vi "Begin.vi"(8 "error in":errorcluster) -> (0 "error out":errorcluster, 2 "Outputs":T1={"West Coast Drive Dev-ref"={"DevStatus"={"status"=FALSE, "code"=0, "source"=""}, "Motors[]"=[], "Square Inputs"=FALSE, "Max Output"=1.0}, "Driver Gamepad"={"Device"=enum."USB 0"}, "Operator Gamepad"={"Device"=enum."USB 0"}, "Shifting Solenoid 1"={"DevStatus"={"status"=FALSE, "code"=0, "source"=""}, "Pneumatics Control Module"=0, "Forward Solenoid Channel"=enum."Invalid", "Reverse Solenoid Channel"=enum."Invalid"}, "Motors"={"Lift Motor 1"={"DeviceStatus"={"status"=FALSE, "code"=0, "source"=""}, "Type"=enum."PWM", "PWM"={"Controller"=enum."Controller 1", "PWM Channel"=enum."PWM 0", "DeadBand"={"Name"="", "maxPositivePwm"=0, "minPositivePwm"=0, "centerPwm"=0, "maxNegativePwm"=0, "minNegativePwm"=0, "angularRange"=0}}, "CAN"={"Device Number"=0, "Control Mode"=enum."Percent VBus", "Semaphore"=refnum, "Max Vout"=0.0, "TalonSRX Control Mode"=enum."Percent VBus"}, "Invert"=FALSE, "TransformRef"=refnum, "InvTransformRef"=refnum}, "Gripper Motor"={"DeviceStatus"={"status"=FALSE, "code"=0, "source"=""}, "Type"=enum."PWM", "PWM"={"Controller"=enum."Controller 1", "PWM Channel"=enum."PWM 0", "DeadBand"={"Name"="", "maxPositivePwm"=0, "minPositivePwm"=0, "centerPwm"=0, "maxNegativePwm"=0, "minNegativePwm"=0, "angularRange"=0}}, "CAN"={"Device Number"=0, "Control Mode"=enum."Percent VBus", "Semaphore"=refnum, "Max Vout"=0.0, "TalonSRX Control Mode"=enum."Percent VBus"}, "Invert"=FALSE, "TransformRef"=refnum, "InvTransformRef"=refnum}, "Lift Motor 2"={"DeviceStatus"={"status"=FALSE, "code"=0, "source"=""}, "Type"=enum."PWM", "PWM"={"Controller"=enum."Controller 1", "PWM Channel"=enum."PWM 0", "DeadBand"={"Name"="", "maxPositivePwm"=0, "minPositivePwm"=0, "centerPwm"=0, "maxNegativePwm"=0, "minNegativePwm"=0, "angularRange"=0}}, "CAN"={"Device Number"=0, "Control Mode"=enum."Percent VBus", "Semaphore"=refnum, "Max Vout"=0.0, "TalonSRX Control Mode"=enum."Percent VBus"}, "Invert"=FALSE, "TransformRef"=refnum, "InvTransformRef"=refnum}}, "Limit Switches"={"SwitchDevRef"={"DevStatus"={"status"=FALSE, "code"=0, "source"=""}, "DIO Channel"=enum."DIO 0", "Controller"=enum."Controller 1", "CntIndex"=enum."Ctr 0", "Normally Closed"=FALSE}, "SwitchDevRef 2"={"DevStatus"={"status"=FALSE, "code"=0, "source"=""}, "DIO Channel"=enum."DIO 0", "Controller"=enum."Controller 1", "CntIndex"=enum."Ctr 0", "Normally Closed"=FALSE}, "SwitchDevRef 3"={"DevStatus"={"status"=FALSE, "code"=0, "source"=""}, "DIO Channel"=enum."DIO 0", "Controller"=enum."Controller 1", "CntIndex"=enum."Ctr 0", "Normally Closed"=FALSE}, "SwitchDevRef 4"={"DevStatus"={"status"=FALSE, "code"=0, "source"=""}, "DIO Channel"=enum."DIO 0", "Controller"=enum."Controller 1", "CntIndex"=enum."Ctr 0", "Normally Closed"=FALSE}}, "Drive Encoders"={"EncoderDevRef"={"DevStatus"={"status"=FALSE, "code"=0, "source"=""}, "EncoderIndex"=enum."Enc 0", "CounterIndex"=enum."Ctr 0", "DistancePerCount"=0.0, "Decoding Type"=enum."1x"}, "EncoderDevRef"={"DevStatus"={"status"=FALSE, "code"=0, "source"=""}, "EncoderIndex"=enum."Enc 0", "CounterIndex"=enum."Ctr 0", "DistancePerCount"=0.0, "Decoding Type"=enum."1x"}}, "Gripper Encoder"={"DevStatus"={"status"=FALSE, "code"=0, "source"=""}, "EncoderIndex"=enum."Invalid", "CounterIndex"=enum."Invalid", "DistancePerCount"=1.0, "Decoding Type"=enum."4x"}, "Lift Potentiometer"={"DevStatus"={"status"=FALSE, "code"=0, "source"=""}, "Controller"=enum."Controller 1", "Analog Channel"=enum."Invalid", "Invert Output"=FALSE}, "Shifting Solenoid 2"={"DevStatus"={"status"=FALSE, "code"=0, "source"=""}, "Pneumatics Control Module"=0, "Forward Solenoid Channel"=enum."Invalid", "Reverse Solenoid Channel"=enum."Invalid"}, "Gyro"={"DevStatus"={"status"=FALSE, "code"=0, "source"=""}, "Analog Module"=enum."Controller 1", "Analog Channel"=enum."AI 1", "Offset"=0.0, "Gain (VoltsPerDegree/Second)"=0.0}, "Buttons"={"Device"=enum."USB 0"}})   [LabVIEW 2014]
doc: "Called before other user functions, this VI is expected to open initial I/O refnums, load in file data, and do all program initialization. Notice that the <B>error out</B> terminal is simply used for data flow. Wiring it to other structures or subVIs ensures that this VI runs first."
uses:
  SubVI/cluster data.ctl
  <vilib>/Rock Robotics/WPI/RobotDrive/WPI_RobotDriveDevRef.ctl
  <vilib>/Rock Robotics/WPI/MotorControl/WPI_MotorControlDeviceRef.ctl
  <vilib>/Rock Robotics/WPI/MotorControl/WPI_MotorControlType.ctl
  <vilib>/Rock Robotics/SystemInterfaces/Typedef/FPGA_TypedefDigitalModule.ctl
  <vilib>/Rock Robotics/SystemInterfaces/DIO/FPGA_DIOPWMChannel.ctl
  <vilib>/Rock Robotics/WPI/PWM/WPI_PWMDeadband.ctl
  <vilib>/Rock Robotics/WPI/CAN/Jaguar/SubVIs/WPI_CANJaguar_ControlMode.ctl
  <vilib>/Rock Robotics/WPI/CAN/TalonSRX/WPI_CANTalonSRX_APIControlMode.ctl
  <vilib>/Rock Robotics/WPI/PWM/WPI_PWMTransform_ConPane.ctl
  <vilib>/Rock Robotics/WPI/Joystick/WPI_JoystickDevRef.ctl
  <vilib>/Rock Robotics/WPI/Joystick/WPI_JoystickDeviceEnum.ctl
  <vilib>/Rock Robotics/WPI/Solenoid/WPI_SolenoidDevRef.ctl
  <vilib>/Rock Robotics/WPI/Solenoid/WPI_SolenoidChannel.ctl
  <vilib>/Rock Robotics/WPI/Switch/WPI_SwitchDevRef.ctl
  <vilib>/Rock Robotics/SystemInterfaces/DIO/FPGA_DIOChannel.ctl
  <vilib>/Rock Robotics/SystemInterfaces/Counter/FPGA_CounterCtrSystemIndex.ctl
  <vilib>/Rock Robotics/WPI/Encoder/WPI_EncoderDevRef.ctl
  <vilib>/Rock Robotics/SystemInterfaces/Encoder/FPGA_EncoderIdx.ctl
  <vilib>/Rock Robotics/WPI/Encoder/WPI_EncoderType.ctl
  <vilib>/Rock Robotics/WPI/Potentiometer/WPI_PotentiometerDevRef.ctl
  <vilib>/Rock Robotics/SystemInterfaces/Typedef/FPGA_TypedefAnalogModule.ctl
  <vilib>/Rock Robotics/SystemInterfaces/AI/FPGA_AIChannel.ctl
  <vilib>/Rock Robotics/WPI/Gyro/WPI_GyroDevRef.ctl
  <vilib>/Rock Robotics/WPI/DriverStation/WPI_DriverStationRobotMode2.ctl
  <vilib>/Rock Robotics/SystemInterfaces/AI/FPGA_AIGyroChannel.ctl
  Robot Global Data.vi
  <vilib>/Rock Robotics/WPI/RobotDrive/WPI_RobotDriveOpen4MotorWithTalon.vi
  <vilib>/Rock Robotics/WPI/Solenoid/WPI_SolenoidOpenSingle.vi
  <vilib>/Rock Robotics/WPI/Counter/WPI_CounterDigitalInputToDigitalSource.vi
  <vilib>/Rock Robotics/WPI/Switch/WPI_SwitchOpenLimit.vi
  <vilib>/Rock Robotics/WPI/MotorControl/WPI_MotorControlOpen Talon.vi
  <vilib>/Rock Robotics/WPI/MotorControl/WPI_MotorControlOpenCANTalonSRX.vi
panel:
  in  "Begin outputs":T1={"West Coast Drive Dev-ref"={"DevStatus"={"status"=FALSE, "code"=0, "source"=""}, "Motors[]"=[], "Square Inputs"=FALSE, "Max Output"=1.0}, "Driver Gamepad"={"Device"=enum."USB 0"}, "Operator Gamepad"={"Device"=enum."USB 0"}, "Shifting Solenoid 1"={"DevStatus"={"status"=FALSE, "code"=0, "source"=""}, "Pneumatics Control Module"=0, "Forward Solenoid Channel"=enum."Invalid", "Reverse Solenoid Channel"=enum."Invalid"}, "Motors"={"Lift Motor 1"={"DeviceStatus"={"status"=FALSE, "code"=0, "source"=""}, "Type"=enum."PWM", "PWM"={"Controller"=enum."Controller 1", "PWM Channel"=enum."Invalid", "DeadBand"={"Name"="", "maxPositivePwm"=0, "minPositivePwm"=0, "centerPwm"=0, "maxNegativePwm"=0, "minNegativePwm"=0, "angularRange"=0}}, "CAN"={"Device Number"=0, "Control Mode"=enum."Percent VBus", "Semaphore"=refnum, "Max Vout"=12.0, "TalonSRX Control Mode"=enum."Percent VBus"}, "Invert"=FALSE, "TransformRef"=refnum, "InvTransformRef"=refnum}, "Gripper Motor"={"DeviceStatus"={"status"=FALSE, "code"=0, "source"=""}, "Type"=enum."PWM", "PWM"={"Controller"=enum."Controller 1", "PWM Channel"=enum."PWM 0", "DeadBand"={"Name"="", "maxPositivePwm"=0, "minPositivePwm"=0, "centerPwm"=0, "maxNegativePwm"=0, "minNegativePwm"=0, "angularRange"=0}}, "CAN"={"Device Number"=0, "Control Mode"=enum."Percent VBus", "Semaphore"=refnum, "Max Vout"=0.0, "TalonSRX Control Mode"=enum."Percent VBus"}, "Invert"=FALSE, "TransformRef"=refnum, "InvTransformRef"=refnum}, "Lift Motor 2"={"DeviceStatus"={"status"=FALSE, "code"=0, "source"=""}, "Type"=enum."PWM", "PWM"={"Controller"=enum."Controller 1", "PWM Channel"=enum."PWM 0", "DeadBand"={"Name"="", "maxPositivePwm"=0, "minPositivePwm"=0, "centerPwm"=0, "maxNegativePwm"=0, "minNegativePwm"=0, "angularRange"=0}}, "CAN"={"Device Number"=0, "Control Mode"=enum."Percent VBus", "Semaphore"=refnum, "Max Vout"=0.0, "TalonSRX Control Mode"=enum."Percent VBus"}, "Invert"=FALSE, "TransformRef"=refnum, "InvTransformRef"=refnum}}, "Limit Switches"={"SwitchDevRef"={"DevStatus"={"status"=FALSE, "code"=0, "source"=""}, "DIO Channel"=enum."DIO 0", "Controller"=enum."Controller 1", "CntIndex"=enum."Ctr 0", "Normally Closed"=FALSE}, "SwitchDevRef 2"={"DevStatus"={"status"=FALSE, "code"=0, "source"=""}, "DIO Channel"=enum."DIO 0", "Controller"=enum."Controller 1", "CntIndex"=enum."Ctr 0", "Normally Closed"=FALSE}, "SwitchDevRef 3"={"DevStatus"={"status"=FALSE, "code"=0, "source"=""}, "DIO Channel"=enum."DIO 0", "Controller"=enum."Controller 1", "CntIndex"=enum."Ctr 0", "Normally Closed"=FALSE}, "SwitchDevRef 4"={"DevStatus"={"status"=FALSE, "code"=0, "source"=""}, "DIO Channel"=enum."DIO 0", "Controller"=enum."Controller 1", "CntIndex"=enum."Ctr 0", "Normally Closed"=FALSE}}, "Drive Encoders"={"EncoderDevRef"={"DevStatus"={"status"=FALSE, "code"=0, "source"=""}, "EncoderIndex"=enum."Enc 0", "CounterIndex"=enum."Ctr 0", "DistancePerCount"=0.0, "Decoding Type"=enum."1x"}, "EncoderDevRef"={"DevStatus"={"status"=FALSE, "code"=0, "source"=""}, "EncoderIndex"=enum."Enc 0", "CounterIndex"=enum."Ctr 0", "DistancePerCount"=0.0, "Decoding Type"=enum."1x"}}, "Gripper Encoder"={"DevStatus"={"status"=FALSE, "code"=0, "source"=""}, "EncoderIndex"=enum."Invalid", "CounterIndex"=enum."Invalid", "DistancePerCount"=1.0, "Decoding Type"=enum."4x"}, "Lift Potentiometer"={"DevStatus"={"status"=FALSE, "code"=0, "source"=""}, "Controller"=enum."Controller 1", "Analog Channel"=enum."Invalid", "Invert Output"=FALSE}, "Shifting Solenoid 2"={"DevStatus"={"status"=FALSE, "code"=0, "source"=""}, "Pneumatics Control Module"=0, "Forward Solenoid Channel"=enum."Invalid", "Reverse Solenoid Channel"=enum."Invalid"}, "Gyro"={"DevStatus"={"status"=FALSE, "code"=0, "source"=""}, "Analog Module"=enum."Controller 1", "Analog Channel"=enum."AI 1", "Offset"=0.0, "Gain (VoltsPerDegree/Second)"=0.0}, "Buttons"={"Device"=enum."USB 0"}}
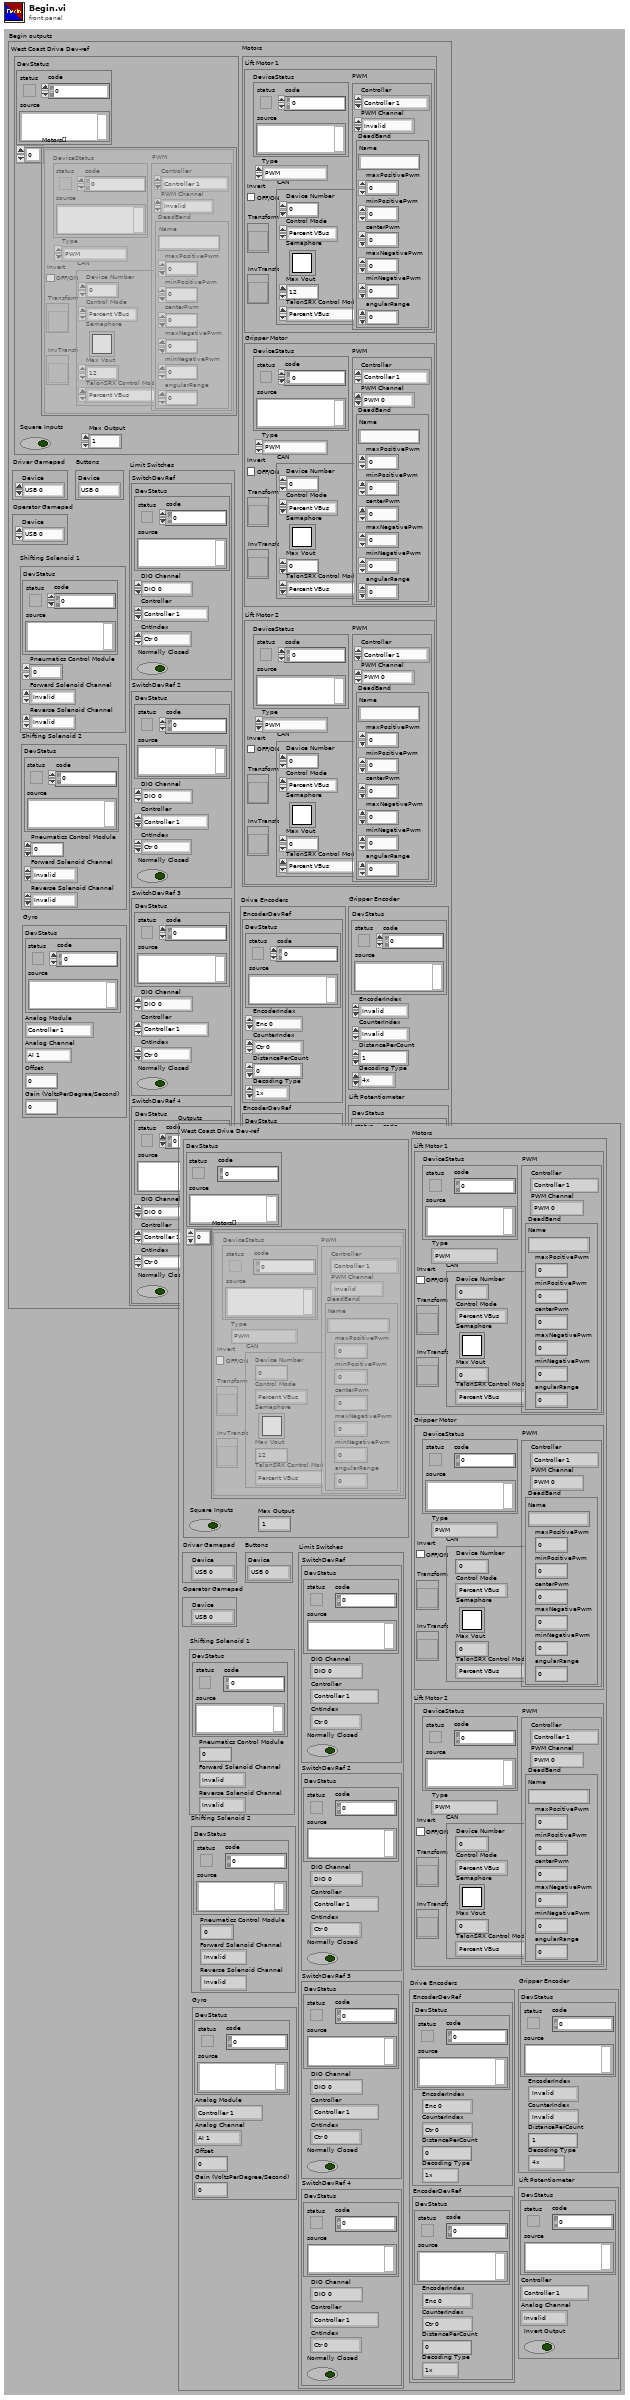
[diagram p1: front panel]
types:
  T1 = typedef "cluster data.ctl" = cluster{"West Coast Drive Dev-ref":T2, "Driver Gamepad":T12, "Operator Gamepad":T12, "Shifting Solenoid 1":T14, "Motors":cluster{"Lift Motor 1":T3, "Gripper Motor":T3, "Lift Motor 2":T3}, "Limit Switches":cluster{"SwitchDevRef":T16, "SwitchDevRef 2":T16, "SwitchDevRef 3":T16, "SwitchDevRef 4":T16}, "Drive Encoders":cluster{"EncoderDevRef":T19, "EncoderDevRef":T19}, "Gripper Encoder":T19, "Lift Potentiometer":T22, "Shifting Solenoid 2":T14, "Gyro":T25, "Buttons":T12}
  T2 = typedef "WPI_RobotDriveDevRef.ctl" = cluster{"DevStatus":errorcluster, "Motors[]":T3[], "Square Inputs":bool, "Max Output":dbl}
  T3 = typedef "WPI_MotorControlDeviceRef.ctl" = cluster{"DeviceStatus":errorcluster, "Type":T4, "PWM":cluster{"Controller":T5, "PWM Channel":T6, "DeadBand":T7}, "CAN":cluster{"Device Number":u8, "Control Mode":T8, "Semaphore":T9, "Max Vout":dbl, "TalonSRX Control Mode":T10}, "Invert":bool, "TransformRef":T11, "InvTransformRef":T11}
  T4 = typedef "WPI_MotorControlType.ctl" = enum16{"PWM", "CAN", "CANTalonSRX"}
  T5 = typedef "FPGA_TypedefDigitalModule.ctl" = enum16{"Controller 1"}
  T6 = typedef "FPGA_DIOPWMChannel.ctl" = enum8{"PWM 0", "PWM 1", "PWM 2", "PWM 3", "PWM 4", "PWM 5", "PWM 6", "PWM 7", "PWM 8", "PWM 9", "PWM MXP 0", "PWM MXP 1", "PWM MXP 2", "PWM MXP 3", "PWM MXP 4", "PWM MXP 5", "PWM MXP 6", "PWM MXP 7", "PWM MXP 8", "PWM MXP 9", "Invalid"}
  T7 = typedef "WPI_PWMDeadband.ctl" = cluster{"Name":string, "maxPositivePwm":i32, "minPositivePwm":i32, "centerPwm":i32, "maxNegativePwm":i32, "minNegativePwm":i32, "angularRange":u16}
  T8 = typedef "WPI_CANJaguar_ControlMode.ctl" = enum8{"Percent VBus", "Current", "Speed", "Position", "Voltage"}
  T9 = typedef "Semaphore RefNum" = refnum<k1>
  T10 = typedef "WPI_CANTalonSRX_APIControlMode.ctl" = enum8{"Percent VBus", "Speed", "Position", "Slave", "Unchanged / Invalid"}
  T11 = typedef "WPI_PWMTransform_ConPane.ctl" = refnum<vi>
  T12 = typedef "WPI_JoystickDevRef.ctl" = cluster{"Device":T13}
  T13 = typedef "WPI_JoystickDeviceEnum.ctl" = enum16{"USB 0", "USB 1", "USB 2", "USB 3", "USB 4", "USB 5"}
  T14 = typedef "WPI_SolenoidDevRef.ctl" = cluster{"DevStatus":errorcluster, "Pneumatics Control Module":u8, "Forward Solenoid Channel":T15, "Reverse Solenoid Channel":T15}
  T15 = typedef "WPI_SolenoidChannel.ctl" = enum8{"Solenoid 0", "Solenoid 1", "Solenoid 2", "Solenoid 3", "Solenoid 4", "Solenoid 5", "Solenoid 6", "Solenoid 7", "Invalid"}
  T16 = typedef "WPI_SwitchDevRef.ctl" = cluster{"DevStatus":errorcluster, "DIO Channel":T17, "Controller":T5, "CntIndex":T18, "Normally Closed":bool}
  T17 = typedef "FPGA_DIOChannel.ctl" = enum8{"DIO 0", "DIO 1", "DIO 2", "DIO 3", "DIO 4", "DIO 5", "DIO 6", "DIO 7", "DIO 8", "DIO 9", "DIO MXP 0", "DIO MXP 1", "DIO MXP 2", "DIO MXP 3", "DIO MXP 4", "DIO MXP 5", "DIO MXP 6", "DIO MXP 7", "DIO MXP 8", "DIO MXP 9", "DIO MXP 10", "DIO MXP 11", "DIO MXP 12", "DIO MXP 13", "DIO MXP 14", "DIO MXP 15", "Invalid"}
  T18 = typedef "FPGA_CounterCtrSystemIndex.ctl" = enum8{"Ctr 0", "Ctr 1", "Ctr 2", "Ctr 3", "Ctr 4", "Ctr 5", "Ctr 6", "Ctr 7", "Invalid"}
  T19 = typedef "WPI_EncoderDevRef.ctl" = cluster{"DevStatus":errorcluster, "EncoderIndex":T20, "CounterIndex":T18, "DistancePerCount":dbl, "Decoding Type":T21}
  T20 = typedef "FPGA_EncoderIdx.ctl" = enum8{"Enc 0", "Enc 1", "Enc 2", "Enc 3", "Enc 4", "Enc 5", "Enc 6", "Enc 7", "Invalid"}
  T21 = typedef "WPI_EncoderType.ctl" = enum16{"1x", "2x", "4x"}
  T22 = typedef "WPI_PotentiometerDevRef.ctl" = cluster{"DevStatus":errorcluster, "Controller":T23, "Analog Channel":T24, "Invert Output":bool}
  T23 = typedef "FPGA_TypedefAnalogModule.ctl" = enum16{"Controller 1"}
  T24 = typedef "FPGA_AIChannel.ctl" = enum8{"AI 0", "AI 1", "AI 2", "AI 3", "AI MXP 0", "AI MXP 1", "AI MXP 2", "AI MXP 3", "Invalid"}
  T25 = typedef "WPI_GyroDevRef.ctl" = cluster{"DevStatus":errorcluster, "Analog Module":T23, "Analog Channel":T24, "Offset":dbl, "Gain (VoltsPerDegree/Second)":dbl}
  T26 = cluster{"Lift Top":T16, "Lift Bottom":T16, "Gripper 1":T16, "Gripper 2":T16}
  T27 = typedef "FPGA_AIGyroChannel.ctl" = enum8{"AI 0", "AI 1", "Invalid"}
  T28 = typedef "WPI_DriverStationRobotMode2.ctl" = enum16{"Autonomous Disabled", "Autonomous Enabled", "Teleop Disabled", "Teleop Enabled", "Disconnected", "Finish", "Test Disabled", "Test Enabled", "Emergency Stopped"}
  T29 = typedef "WPI_DigitalInputDevRef.ctl" = cluster{"DevStatus":errorcluster, "DIO Channel":T17, "Controller":T5}
  T30 = typedef "FPGA_CounterEncoderSourceConvertionLVSourceType.ctl" = cluster{"DevStatus":errorcluster, "AnalogTriggerMode?":bool, "DigitalMode":cluster{"Controller":T5, "DIO Channel":T31}, "AnalogTriggerMode":cluster{"AnalogTriggerIndex":T32, "OutputType":T33}}
  T31 = typedef "FPGA_DIODigitalSourceChannel.ctl" = enum8{"DIO 0", "DIO 1", "DIO 2", "DIO 3", "DIO 4", "DIO 5", "DIO 6", "DIO 7", "DIO 8", "DIO 9", "DIO MXP 0", "DIO MXP 1", "DIO MXP 2", "DIO MXP 3", "DIO MXP 4", "DIO MXP 5", "DIO MXP 6", "DIO MXP 7", "DIO MXP 8", "DIO MXP 9", "DIO MXP 10", "DIO MXP 11", "DIO MXP 12", "DIO MXP 13", "DIO MXP 14", "DIO MXP 15", "Disabled"}
  T32 = typedef "FPGA_AnalogTriggerIndex.ctl" = enum8{"Trig 0", "Trig 1", "Trig 2", "Trig 3", "Trig 4", "Trig 5", "Trig 6", "Trig 7", "Invalid"}
  T33 = typedef "FPGA_AnalogTriggerOutType.ctl" = enum16{"InWindow", "TriggerState", "Rising", "Falling"}
  T34 = cluster{"EncoderDevRef":T19, "EncoderDevRef":T19}
  T35 = cluster{"MotorControlDeviceRef":T3, "MotorControlDeviceRef":T3, "MotorControlDeviceRef":T3}
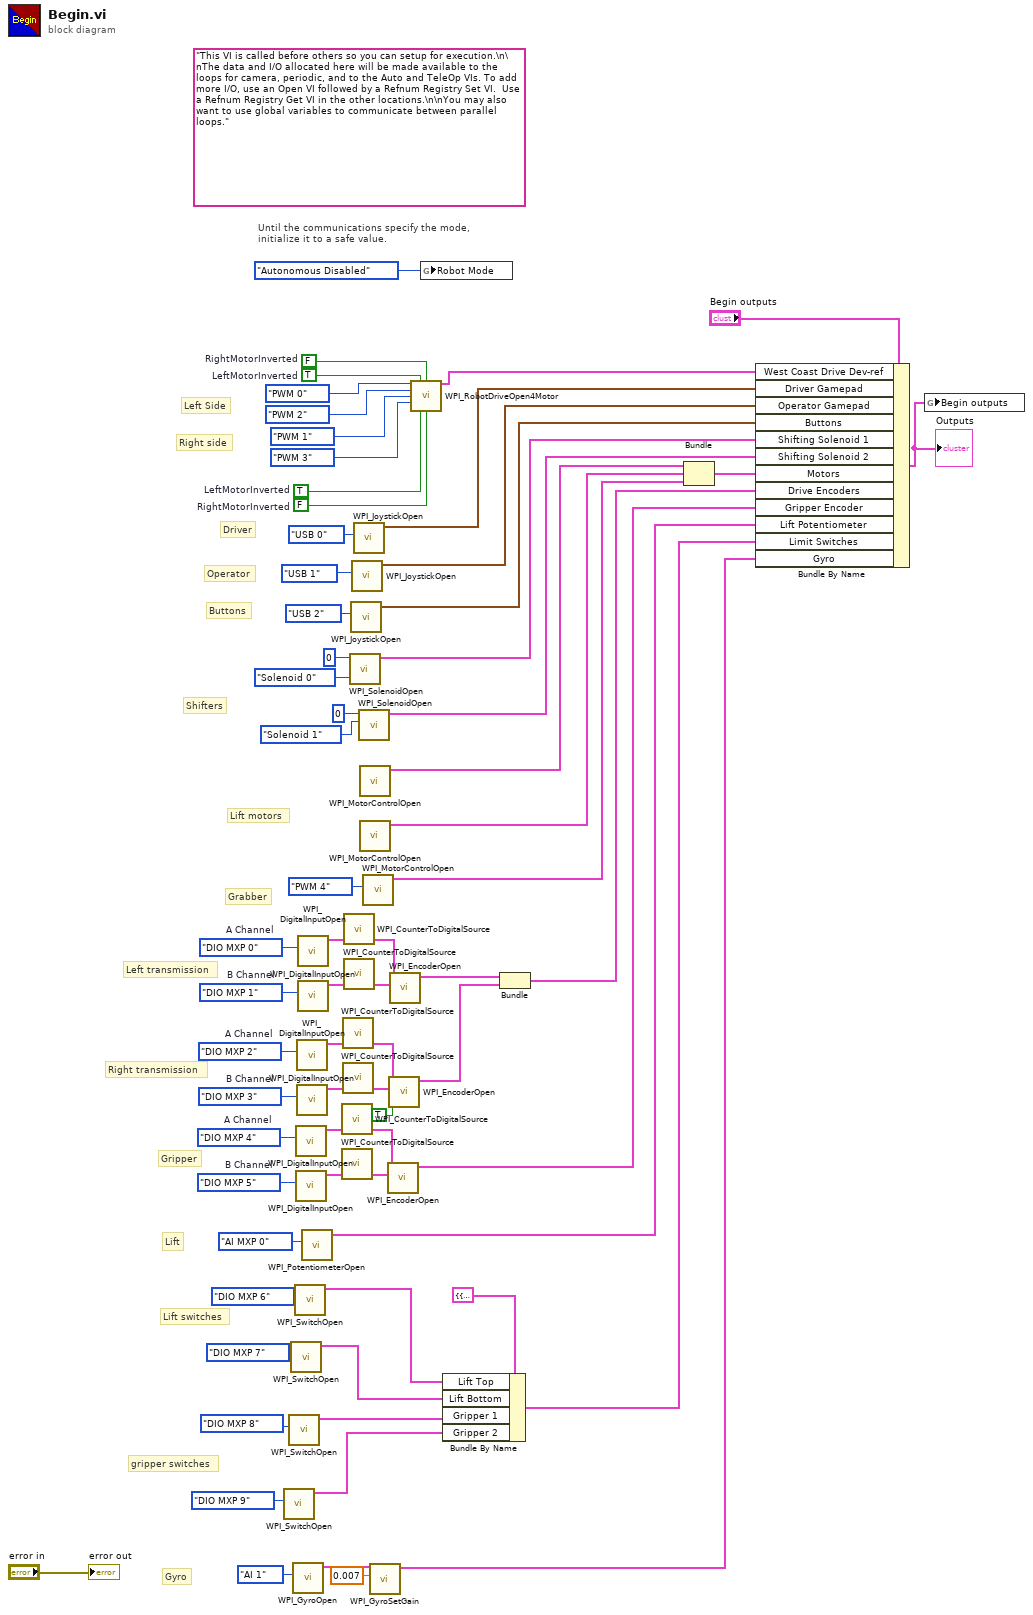
[diagram p0: block diagram]
diagram:
  w36 = FPGA_DIOChannel."DIO MXP 5"  # B Channel
  w35 = FPGA_DIOChannel."DIO MXP 4"  # A Channel
  w42 = FPGA_DIOChannel."DIO MXP 3"  # B Channel
  w41 = FPGA_DIOChannel."DIO MXP 2"  # A Channel
  w48 = FPGA_DIOChannel."DIO MXP 1"  # B Channel
  w47 = FPGA_DIOChannel."DIO MXP 0"  # A Channel
  w61 = FALSE  # RightMotorInverted
  w60 = TRUE  # LeftMotorInverted
  (unwired) "This VI is called before others so you can setup for execution.\n\nThe data and I/O allocated here will be made available to the loops for camera, periodic, and to the Auto and TeleOp VIs. To add more I/O, use an Open VI followed by a Refnum Registry Set VI.  Use a Refnum Registry Get VI in the other locations.\n\nYou may also want to use global variables to communicate between parallel loops."
  w67 = TRUE  # LeftMotorInverted
  w66 = FALSE  # RightMotorInverted
  # "Buttons"
  # "Gyro"
  # "gripper switches"
  # "Lift switches"
  # "Gripper"
  # "Lift"
  # "Right transmission"
  # "Left transmission"
  # "Grabber"
  # "Lift motors"
  # "Shifters"
  # "Operator"
  # "Driver"
  # "Right side"
  # "Left Side"
  # "Until the communications specify the mode,\ninitialize it to a safe value."
  n1 = call-poly <vilib>:"WPI_SwitchOpen.vi"("DIO Channel"=FPGA_DIOChannel."DIO MXP 9") -> ("SwitchDevRef"=w22:T16)  [unwired: 9 in, 1 out]
  n2 = call-poly <vilib>:"WPI_SwitchOpen.vi"("DIO Channel"=FPGA_DIOChannel."DIO MXP 8") -> ("SwitchDevRef"=w16:T16)  [unwired: 9 in, 1 out]
  n3 = call-poly <vilib>:"WPI_SwitchOpen.vi"("DIO Channel"=FPGA_DIOChannel."DIO MXP 7") -> ("SwitchDevRef"=w23:T16)  [unwired: 9 in, 1 out]
  n4 = call <vilib>:"WPI_GyroOpen.vi"("Analog Channel"=FPGA_AIGyroChannel."AI 1") -> ("GyroDevRef"=w5:T25)  [unwired: 8 in, 2 out]
  n5 = call-poly <vilib>:"WPI_SwitchOpen.vi"("DIO Channel"=FPGA_DIOChannel."DIO MXP 6") -> ("SwitchDevRef"=w24:T16)  [unwired: 9 in, 1 out]
  n6 = call <vilib>:"WPI_DigitalInputOpen.vi"("DIO Channel"=w35) -> ("DigitalInputDevRef"=w32:T29)  [unwired: 2 in, 8 out]
  n7 = call <vilib>:"WPI_DigitalInputOpen.vi"("DIO Channel"=w36) -> ("DigitalInputDevRef"=w33:T29)  [unwired: 2 in, 8 out]
  n8 = call <vilib>:"WPI_DigitalInputOpen.vi"("DIO Channel"=w41) -> ("DigitalInputDevRef"=w38:T29)  [unwired: 2 in, 8 out]
  n9 = call <vilib>:"WPI_DigitalInputOpen.vi"("DIO Channel"=w42) -> ("DigitalInputDevRef"=w39:T29)  [unwired: 2 in, 8 out]
  n10 = call <vilib>:"WPI_DigitalInputOpen.vi"("DIO Channel"=w47) -> ("DigitalInputDevRef"=w44:T29)  [unwired: 2 in, 8 out]
  n11 = call <vilib>:"WPI_DigitalInputOpen.vi"("DIO Channel"=w48) -> ("DigitalInputDevRef"=w45:T29)  [unwired: 2 in, 8 out]
  n12 = call <vilib>:"WPI_PotentiometerOpen.vi"("Analog Channel"=FPGA_AIChannel."AI MXP 0") -> ("PotDevRef"=w17:T22)  [unwired: 9 in, 1 out]
  n13 = call-poly <vilib>:"WPI_CounterToDigitalSource.vi"("DigitalInputDevRef"=w32) -> ("Digital Source"=w31:T30)  [unwired: 6 out]
  n14 = call-poly <vilib>:"WPI_CounterToDigitalSource.vi"("DigitalInputDevRef"=w33) -> ("Digital Source"=w34:T30)  [unwired: 6 out]
  n15 = call-poly <vilib>:"WPI_CounterToDigitalSource.vi"("DigitalInputDevRef"=w38) -> ("Digital Source"=w37:T30)  [unwired: 6 out]
  n16 = call-poly <vilib>:"WPI_CounterToDigitalSource.vi"("DigitalInputDevRef"=w39) -> ("Digital Source"=w40:T30)  [unwired: 6 out]
  n17 = call-poly <vilib>:"WPI_CounterToDigitalSource.vi"("DigitalInputDevRef"=w44) -> ("Digital Source"=w43:T30)  [unwired: 6 out]
  n18 = call-poly <vilib>:"WPI_CounterToDigitalSource.vi"("DigitalInputDevRef"=w45) -> ("Digital Source"=w46:T30)  [unwired: 6 out]
  n19 = call-poly <vilib>:"WPI_SolenoidOpen.vi"("Solenoid Channel"=WPI_SolenoidChannel."Solenoid 0" ("Forward Solenoid Channel"), "Pneumatics Control Module (0)"=u8 0) -> ("SolenoidDevRef"=w52:T14)  [unwired: 8 in, 1 out]
  n20 = call <vilib>:"WPI_JoystickOpen.vi"("JoystickDevice"=WPI_JoystickDeviceEnum."USB 2") -> ("JoystickDevRef"=w1:T12)  [unwired: 10 in]
  n21 = call <vilib>:"WPI_JoystickOpen.vi"("JoystickDevice"=WPI_JoystickDeviceEnum."USB 1") -> ("JoystickDevRef"=w58:T12)  [unwired: 10 in]
  n22 = call <vilib>:"WPI_JoystickOpen.vi"("JoystickDevice"=WPI_JoystickDeviceEnum."USB 0") -> ("JoystickDevRef"=w57:T12)  [unwired: 10 in]
  n23 = call-poly <vilib>:"WPI_SolenoidOpen.vi"("Solenoid Channel"=WPI_SolenoidChannel."Solenoid 1" ("Reverse Solenoid Channel"), "Pneumatics Control Module (0)"=u8 0) -> ("SolenoidDevRef"=w12:T14)  [unwired: 8 in, 1 out]
  n24 = call-poly <vilib>:"WPI_MotorControlOpen.vi"() -> ("MotorControlDeviceRef"=w50:T3)  [unwired: 10 in, 1 out]
  n25 = call-poly <vilib>:"WPI_MotorControlOpen.vi"() -> ("MotorControlDeviceRef"=w49:T3)  [unwired: 10 in, 1 out]
  n26 = call-poly <vilib>:"WPI_MotorControlOpen.vi"("PWM Channel"=FPGA_DIOPWMChannel."PWM 4") -> ("MotorControlDeviceRef"=w8:T3)  [unwired: 9 in, 1 out]
  n27 = call <vilib>:"WPI_GyroSetGain.vi"("Gain (VoltsPerDegree/Second)"=0.007, "GyroDevRef"=w5) -> ("GyroDevRef"=w4:T25)  [unwired: 8 in, 1 out]
  n28 = call <vilib>:"WPI_EncoderOpen.vi"("BSource"=w34, "ASource"=w31) -> ("EncoderDevRef"=w18:T19)  [unwired: 6 in, 3 out]
  n29 = call <vilib>:"WPI_EncoderOpen.vi"("Invert Direction (False)"=TRUE, "BSource"=w40, "ASource"=w37) -> ("EncoderDevRef"=w20:T19)  [unwired: 5 in, 3 out]
  n30 = call <vilib>:"WPI_EncoderOpen.vi"("BSource"=w46, "ASource"=w43) -> ("EncoderDevRef"=w21:T19)  [unwired: 6 in, 3 out]
  n31 = call-poly <vilib>:"WPI_RobotDriveOpen4Motor.vi"("Rear Left Motor"=FPGA_DIOPWMChannel."PWM 0", "Rear Left Motor Inverted"=w67, "Rear Right Motor Inverted"=w66, "Rear Right Motor"=FPGA_DIOPWMChannel."PWM 2", "Front Left Motor"=FPGA_DIOPWMChannel."PWM 1", "Front Right Motor"=FPGA_DIOPWMChannel."PWM 3", "Front Left Motor Inverted"=w60, "Front Right Motor Inverted"=w61) -> ("RobotDriveDevRef"=w59:T2)  [unwired: 6 in, 1 out]
  n32 = global write "Robot Global Data.vi" "Robot Mode"(WPI_DriverStationRobotMode2."Autonomous Disabled" ("Robot Mode")) -> ()
  n33 = Bundle By Name(cluster=T26 {"Lift Top"={"DevStatus"={"status"=FALSE, "code"=0, "source"=""}, "DIO Channel"=enum."Invalid", "Controller"=enum."Controller 1", "CntIndex"=enum."Invalid", "Normally Closed"=FALSE}, "Lift Bottom"={"DevStatus"={"status"=FALSE, "code"=0, "source"=""}, "DIO Channel"=enum."Invalid", "Controller"=enum."Controller 1", "CntIndex"=enum."Invalid", "Normally Closed"=FALSE}, "Gripper 1"={"DevStatus"={"status"=FALSE, "code"=0, "source"=""}, "DIO Channel"=enum."Invalid", "Controller"=enum."Controller 1", "CntIndex"=enum."Invalid", "Normally Closed"=FALSE}, "Gripper 2"={"DevStatus"={"status"=FALSE, "code"=0, "source"=""}, "DIO Channel"=enum."Invalid", "Controller"=enum."Controller 1", "CntIndex"=enum."Invalid", "Normally Closed"=FALSE}} ("Limit Switches"), "Lift Top"=w24, "Lift Bottom"=w23, "Gripper 1"=w16, "Gripper 2"=w22) -> (w15:T26)
  n34 = Bundle("EncoderDevRef"=w21, "EncoderDevRef"=w20) -> (w19:T34)  [unwired: 1 in]
  n35 = Bundle("MotorControlDeviceRef"=w50, "MotorControlDeviceRef"=w49, "MotorControlDeviceRef"=w8) -> (w13:T35)  [unwired: 1 in]
  n36 = Bundle By Name(cluster="Begin outputs", "West Coast Drive Dev-ref"=w59, "Driver Gamepad"=w57, "Operator Gamepad"=w58, "Buttons"=w1, "Shifting Solenoid 1"=w52, "Shifting Solenoid 2"=w12, "Motors"=w13, "Drive Encoders"=w19, "Gripper Encoder"=w18, "Lift Potentiometer"=w17, "Limit Switches"=w15, "Gyro"=w4) -> (w11:T1)
  "Outputs" <- w11
  n37 = global write "Robot Global Data.vi" "Begin outputs"(w11) -> ()
  "error out" <- "error in"
